vi "Robot Global Data.vi"() -> ()   [LabVIEW 2017]
doc: "This global VI can contain as many global variables as you need. To create a global variable, place a control on the panel, give it a good name. To read or write to it from a VI, drag the icon to the diagram of that VI. You can also drag from the project. Click on the node to change which global you access. You shouldn't have multiple locations writing to a global or it will cause a race-condition."
uses:
  <vilib>/Rock Robotics/WPI/Camera/WPI_CameraImageSize.ctl
  <vilib>/Rock Robotics/WPI/DriverStation/WPI_DriverStationRobotMode2.ctl
  Shared/AutoRoutineSelector.ctl
  Shared/2CubeOption.ctl
panel:
  in  "TryA3Cube":bool
  in  "TwoCubeSelectors":T1[](array[typedef])=[enum."Nothing", enum."Nothing", enum."Nothing", enum."Nothing"]
  in  "NotPurePursuit":bool
  in  "Position":u32=1
  in  "Routine":T2
  in  "Duration":dbl
  in  "Left Joystick":dbl
  in  "Right Joystick":dbl
  in  "Robot Mode":T3
  in  "image size":T4=enum."320x240"
  in  "Enable Vision":bool
  # "AUTO ROUTINE"
  # "Switch Other Close"
  # "SW NC"
  # "SCC"
  # "SCNC"
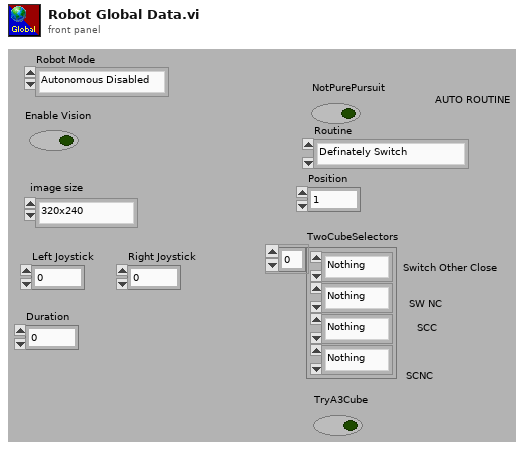
[diagram p1: front panel]
types:
  T1 = typedef "2CubeOption.ctl" = enum16{"Nothing", "Switch", "Scale"}
  T2 = typedef "AutoRoutineSelector.ctl" = enum16{"Definately Switch", "Definately Scale", "Switch if in front, else scale", "Scale if in front, else switch", "Switch if in front, else cross line", "Scale if in front, else cross line", "Drive across line"}
  T3 = typedef "WPI_DriverStationRobotMode2.ctl" = enum16{"Autonomous Disabled", "Autonomous Enabled", "Teleop Disabled", "Teleop Enabled", "Disconnected", "Finish", "Test Disabled", "Test Enabled", "Emergency Stopped"}
  T4 = typedef "WPI_CameraImageSize.ctl" = enum16{"640x480", "320x240", "160x120", "Custom"}
diagram:
